vi "Error to State.vi"(6 "Opposite End (T)":bool=TRUE, 8 "error in (no error)":errorcluster, 9 "Error Code":i32, 10 "Element":string, 11 "queue":refnum<queue>) -> (0 "error out":errorcluster, 3 "queue out":refnum<queue>)   [LabVIEW 2011]
doc: "Checks for an error (or warning) code, and if found enqueues the specified element on the queue.\n\n\nVersion 1.1 - 5/1/2010\n\nPhaeron, Inc.\nwww.phaeron.com\ninfo@phaeron.com"
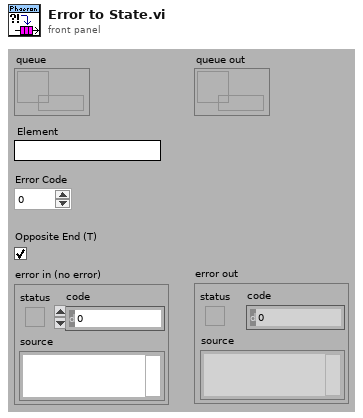
[diagram p1: front panel]
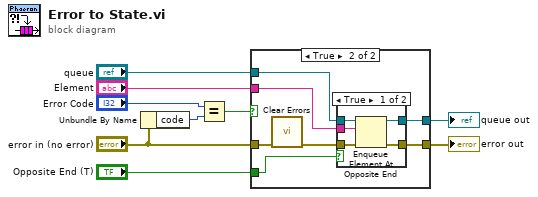
[diagram p0: block diagram]
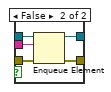
[diagram p3: hidden frame]
diagram:
  n1 = Unbundle By Name("error in (no error)") -> ("code"=w9:i32)
  n2 = Equal?(x="Error Code", y=w9) -> (x = y?=w4:bool)
  n3 = case shown="True" w4 {
    tunnel: "error in (no error)" -> [w11 w18]
    tunnel: [w11 w17] -> w6
    tunnel: "queue" -> [w10 w16]
    tunnel: "Element" -> [_ w14]
    tunnel: [w10 w13] -> w2
    tunnel: "Opposite End (T)" -> [_ w12]
    frame False {
    }
    frame True {
      n4 = call <vilib>:"Clear Errors.vi"("error in (no error)"=w18) -> ("error out"=w15:errorcluster)  [unwired: 6 in]
      n5 = case shown="True" w12 {
        tunnel: [w23 w28] -> w17
        tunnel: w16 -> [w22 w27]
        tunnel: w15 -> [w21 w26]
        tunnel: w14 -> [w20 w25]
        tunnel: [w19 w24] -> w13
        frame True {
          n6 = Enqueue Element At Opposite End(queue=w22, element=w20, error in (no error)=w21) -> (queue out=w19:refnum<queue>, error out=w23:errorcluster)  [unwired: 1 in, 1 out]
        }
        frame False {
          n7 = Enqueue Element(queue=w27, element=w25, error in (no error)=w26) -> (queue out=w24:refnum<queue>, error out=w28:errorcluster)  [unwired: 1 in, 1 out]
        }
      }
    }
  }
  "error out" <- w6
  "queue out" <- w2
